vi "Utility_Initialization.vi"(8 "error in (no error)":errorcluster, 10 "path":path, 11 "Fluidofinterest":string="PROPANE.FLD") -> (0 "error out":errorcluster, 2 "name out":string, 3 "Mixure Cluster out":T1)   [LabVIEW 2016]
doc: "Initializes Refprop by running SETUP pojn a given fluid of interest\n\nPlease feel free to contact me if you have any questions .\nMy mail:ken_pop@tom.com yan.ding@jci.com"
uses:
  Ctl/hrf_enum_d.ctl
  Ctl/Mixture Composition cluster_d.ctl
panel:
  out "hmx_pathout":path
  in  "ReferenceState(hrf)":T2
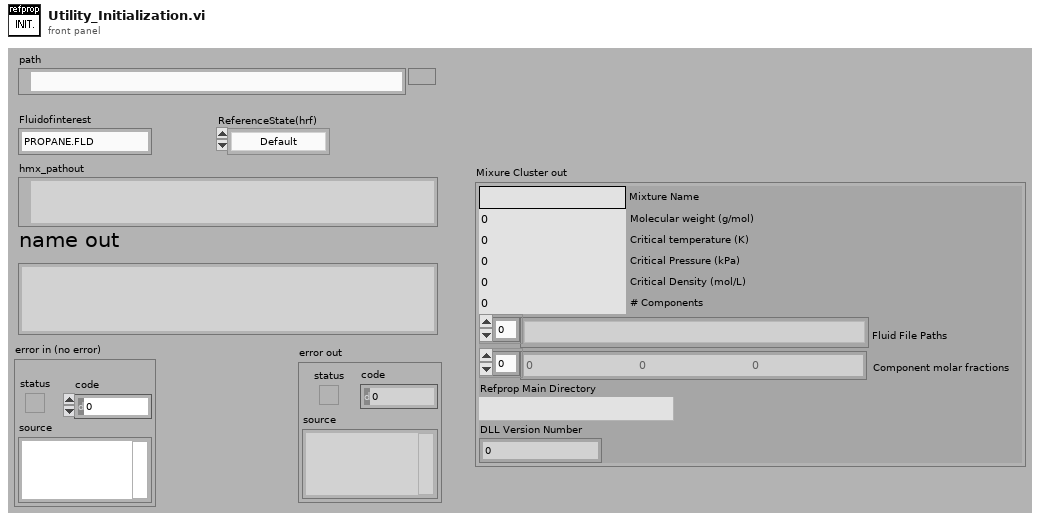
[diagram p1: front panel]
types:
  T1 = typedef "Mixture Composition cluster_d.ctl" = cluster{"Mixture Name":string, "Molecular weight (g/mol)":dbl, "Critical temperature (K)":dbl, "Critical Pressure (kPa)":dbl, "Critical Density (mol/L)":dbl, "# Components":i32, "Fluid File Paths":path[], "Component molar fractions":dbl[], "Refprop Main Directory":path, "DLL Version Number":dbl}
  T2 = typedef "hrf_enum_d.ctl" = enum16{"Default", "ASHRAE", "IIR"}
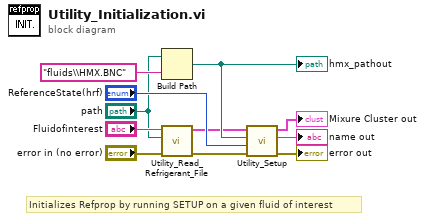
[diagram p0: block diagram]
diagram:
  # "Initializes Refprop by running SETUP on a given fluid of interest"
  n1 = Build Path(base path="path", name or relative path="fluids\\HMX.BNC" ("名称或相对路径")) -> (appended path=w6:path)
  "hmx_pathout" <- w6
  n2 = call "Utility_Read_Refrigerant_File.vi"("error in (no error)"="error in (no error)", "Refprop Main Directory"="path", "Refrigerant File"="Fluidofinterest") -> ("error out"=w10:errorcluster, "Mixure Cluster"=w1:T1)  [unwired: 5 in]
  n3 = call "Utility_Setup.vi"("error in (no error)"=w10, "Reference State (hrf)"="ReferenceState(hrf)", "Path to Mixture file (hfmix)"=w6, "Mixure Cluster in"=w1) -> ("error out"=→"error out":errorcluster, "name out"=→"name out":string, "Mixure Cluster out"=→"Mixure Cluster out":T1)  [unwired: 3 in]
